vi "Size to Rectangle.vi"(1 "Size":cluster{"Width":u32, "Height":u32}) -> (0 "rect":T1)   [LabVIEW 2009]
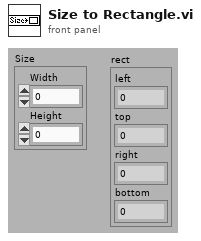
[diagram p1: front panel]
types:
  T1 = cluster{"left":i16, "top":i16, "right":i16, "bottom":i16}
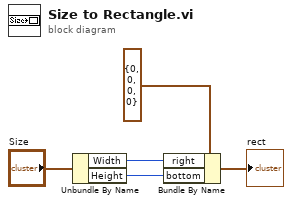
[diagram p0: block diagram]
diagram:
  n1 = Unbundle By Name("Size") -> ("Width"=w3:u32, "Height"=w2:u32)
  n2 = Bundle By Name(cluster=T1 {"left"=0, "top"=0, "right"=0, "bottom"=0} ("rect"), "right"=w3, "bottom"=w2) -> (→"rect":T1)
